vi "Get Debug Flags.vi"(11 "Interface in":refnum<class "Interface.lvclass">) -> (2 "FIFO Debug Flags":refnum<class "FIFO Flags.lvclass">, 3 "Interface out":refnum<class "Interface.lvclass">)   [LabVIEW 2017, in "DSF Core.lvlib" / "Interface.lvclass"]
uses:
  Interface.lvclass
  Debug/FIFO Flags/FIFO Flags.lvclass
  Interface.lvclass/Interface.ctl
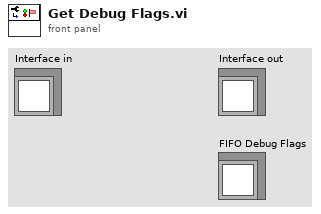
[diagram p1: front panel]
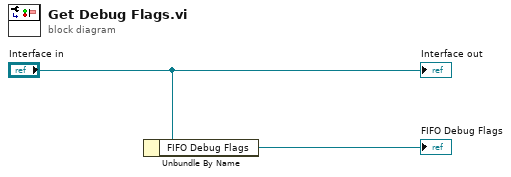
[diagram p0: block diagram]
diagram:
  n1 = Unbundle By Name("Interface in") -> ("FIFO Debug Flags"=→"FIFO Debug Flags":refnum<class "FIFO Flags.lvclass">)
  "Interface out" <- "Interface in"
